vi "real time object finder single cam 4 way v2.1 EJA 09 19 2016.vi"() -> ()   [LabVIEW 2013]
doc: "The Low-Level Grab VI acquires images continuously and displays the images in an image control using low-level acquisition VIs. A grab is appropriate for high-speed applications in which you need to process only one image at a time."
uses:
  <vilib>/userdefined/High Color/IMAQdx.ctl
  <vilib>/vision/driver/IMAQdx.llb/IMAQdx Buffer Number Mode.ctl
  <vilib>/Utility/file.llb/Write To Spreadsheet File (I64).vi
  <vilib>/vision/driver/NI_Vision_Acquisition_Software.lvlib
  <resource>/objmgr/imaqdx.rc
  <vilib>/Analysis/NI_AALBase.lvlib
panel:
  in  "Rectangle":T1
  in  "fish size":i32=200
  out "y position histogram":T2(graph)={"X Values"=[445.05, 445.15, 445.25, 445.35, 445.45, 445.55, 445.65, 445.75, 445.85, 445.95], "Histogram: h(x)"=[229, 0, 0, 0, 0, 0, 0, 0, 0, 272]}
  out "x position histogram":T2(graph)={"X Values"=[585.0, 585.0, 585.0, 585.0, 585.0, 585.0, 585.0, 585.0, 585.0, 585.0], "Histogram: h(x)"=[0, 0, 0, 0, 0, 0, 0, 0, 0, 501]}
  in  "histogram \nbins":i32=10
  in  "always save\non stop\nimaging":bool=TRUE
  in  "acquisition \ntime (s)":i32=10
  in  "save for a \ndesignated \nperiod":bool=TRUE
  out "trajectory":cluster{i32[], i32[]}(graph)={[585, 585, 585, 585, 585, 585, 585, 585, 585, 585, 585, 585, 585, 585, 585, 585, 585, 585, 585, 585, 585, 585, 585, 585, 585, 585, 585, 585, 585, 585, 585, 585, 585, 585, 585, 585, 585, 585, 585, 585, 585, 585, 585, 585, 585, 585, 585, 585, 585, 585, 585, 585, 585, 585, 585, 585, 585, 585, 585, 585, 585, 585, 585, 585, 585, 585, 585, 585, 585, 585, 585, 585, 585, 585, 585, 585, 585, 585, 585, 585, 585, 585, 585, 585, 585, 585, 585, 585, 585, 585, 585, 585, 585, 585, 585, 585, 585, 585, 585, 585, 585, 585, 585, 585, 585, 585, 585, 585, 585, 585, 585, 585, 585, 585, 585, 585, 585, 585, 585, 585, 585, 585, 585, 585, 585, 585, 585, 585, 585, 585, 585, 585, 585, 585, 585, 585, 585, 585, 585, 585, 585, 585, 585, 585, 585, 585, 585, 585, 585, 585, 585, 585, 585, 585, 585, 585, 585, 585, 585, 585, 585, 585, 585, 585, 585, 585, 585, 585, 585, 585, 585, 585, 585, 585, 585, 585, 585, 585, 585, 585, 585, 585, 585, 585, 585, 585, 585, 585, 585, 585, 585, 585, 585, 585, 585, 585, 585, 585, 585, 585, 585, 585, 585, 585, 585, 585, 585, 585, 585, 585, 585, 585, 585, 585, 585, 585, 585, 585, 585, 585, 585, 585, 585, 585, 585, 585, 585, 585, 585, 585, 585, 585, 585, 585, 585, 585, 585, 585, 585, 585, 585, 585, 585, 585, 585, 585, 585, 585, 585, 585, 585, 585, 585, 585, 585, 585, 585, 585, 585, 585, 585, 585, 585, 585, 585, 585, 585, 585, 585, 585, 585, 585, 585, 585, 585, 585, 585, 585, 585, 585, 585, 585, 585, 585, 585, 585, 585, 585, 585, 585, 585, 585, 585, 585, 585, 585, 585, 585, 585, 585, 585, 585, 585, 585, 585, 585, 585, 585, 585, 585, 585, 585, 585, 585, 585, 585, 585, 585, 585, 585, 585, 585, 585, 585, 585, 585, 585, 585, 585, 585, 585, 585, 585, 585, 585, 585, 585, 585, 585, 585, 585, 585, 585, 585, 585, 585, 585, 585, 585, 585, 585, 585, 585, 585, 585, 585, 585, 585, 585, 585, 585, 585, 585, 585, 585, 585, 585, 585, 585, 585, 585, 585, 585, 585, 585, 585, 585, 585, 585, 585, 585, 585, 585, 585, 585, 585, 585, 585, 585, 585, 585, 585, 585, 585, 585, 585, 585, 585, 585, 585, 585, 585, 585, 585, 585, 585, 585, 585, 585, 585, 585, 585, 585, 585, 585, 585, 585, 585, 585, 585, 585, 585, 585, 585, 585, 585, 585, 585, 585, 585, 585, 585, 585, 585, 585, 585, 585, 585, 585, 585, 585, 585, 585, 585, 585, 585, 585, 585, 585, 585, 585, 585, 585, 585, 585, 585, 585, 585, 585, 585, 585, 585, 585, 585, 585, 585, 585, 585, 585, 585, 585, 585, 585, 585, 585, 585, 585, 585, 585, 585, 585, 585, 585, 585, 585, 585, 585, 585, 585, 585, 585, 585, 585, 585, 585, 585, 585, 585, 585, 585, 585], [446, 446, 446, 445, 446, 445, 446, 446, 446, 446, 446, 445, 445, 446, 445, 446, 445, 446, 446, 446, 445, 445, 446, 446, 445, 445, 446, 445, 446, 445, 445, 445, 445, 445, 446, 446, 445, 445, 445, 446, 446, 445, 445, 445, 446, 446, 446, 445, 446, 446, 446, 446, 446, 445, 446, 446, 445, 446, 445, 446, 445, 445, 445, 446, 445, 446, 446, 446, 446, 446, 445, 445, 445, 445, 446, 445, 445, 445, 445, 446, 445, 446, 446, 446, 446, 446, 446, 445, 445, 446, 445, 445, 445, 445, 445, 445, 445, 445, 446, 446, 446, 445, 446, 445, 446, 445, 445, 446, 446, 446, 446, 445, 446, 445, 446, 445, 445, 445, 446, 446, 445, 445, 446, 445, 446, 445, 446, 446, 445, 446, 446, 445, 445, 445, 446, 445, 446, 445, 445, 446, 446, 445, 445, 446, 445, 446, 446, 446, 446, 445, 445, 446, 445, 445, 446, 445, 445, 445, 445, 445, 445, 446, 446, 445, 446, 445, 446, 446, 445, 446, 445, 446, 446, 445, 446, 446, 445, 446, 445, 446, 446, 446, 445, 446, 445, 446, 446, 445, 446, 445, 446, 445, 446, 445, 446, 445, 445, 445, 446, 445, 446, 446, 446, 445, 445, 446, 446, 446, 445, 446, 445, 446, 445, 446, 446, 446, 446, 446, 446, 446, 446, 445, 446, 445, 445, 445, 446, 445, 445, 446, 445, 445, 446, 446, 446, 445, 446, 445, 446, 446, 446, 445, 445, 445, 446, 446, 446, 445, 445, 445, 446, 445, 445, 446, 445, 445, 446, 446, 445, 445, 446, 446, 446, 446, 446, 446, 446, 446, 446, 446, 445, 446, 445, 445, 445, 446, 445, 446, 445, 446, 445, 445, 445, 446, 446, 446, 445, 446, 445, 445, 445, 446, 446, 446, 446, 445, 446, 446, 446, 445, 445, 445, 446, 446, 446, 446, 445, 446, 445, 446, 446, 445, 446, 446, 446, 446, 445, 446, 445, 445, 445, 446, 446, 445, 446, 446, 445, 446, 446, 446, 446, 446, 446, 445, 446, 446, 445, 446, 446, 445, 446, 445, 446, 446, 446, 446, 445, 446, 446, 446, 446, 446, 445, 446, 446, 446, 446, 446, 446, 446, 445, 445, 445, 445, 445, 445, 445, 446, 445, 446, 446, 446, 446, 445, 446, 446, 445, 445, 445, 445, 445, 446, 445, 445, 445, 445, 446, 446, 445, 445, 445, 445, 446, 445, 446, 446, 446, 446, 445, 445, 445, 445, 445, 446, 445, 445, 446, 445, 445, 446, 446, 446, 445, 446, 445, 446, 445, 446, 445, 446, 445, 446, 445, 446, 446, 445, 446, 445, 446, 445, 445, 446, 446, 445, 445, 445, 445, 445, 446, 445, 445, 446, 446, 446, 446, 445, 446, 445, 446, 446, 446, 445, 445, 446, 445, 446, 446, 446, 446, 445, 446, 445, 446, 446, 445, 446, 446, 445, 445, 446, 446, 445, 446, 446, 446, 445, 446, 446, 446, 445, 445, 445, 446, 445, 446, 446, 446, 446, 445, 445, 446, 445, 445, 446, 445, 446, 446, 446, 446, 446, 445]}
  in  "save\nlast\nimage":bool=TRUE
  in  "stop no save":bool
  out "date stub assigned":string="_2016Y_10M_31D_13h_16m_16s"
  in  "Acquire\ndata":bool
  in  "Experimental stub":string="danio02"
  out "Saving":bool
  in  "save data":bool
  in  "save path":path=path "C:/danio_tracking/danio02_10_28_2016"
  in  "number\nformat (%.6f)":string="%.6f"
  in  "Marker\nText color":u32(colorbox)=16711680
  out "Multiplot":cluster{cluster{dbl, i32}[]}[](graph)=[{[{0.0, 585}, {0.02, 585}, {0.04, 585}, {0.06, 585}, {0.08, 585}, {0.1, 585}, {0.12, 585}, {0.14, 585}, {0.16, 585}, {0.18, 585}, {0.2, 585}, {0.22, 585}, {0.24, 585}, {0.26, 585}, {0.281, 585}, {0.301, 585}, {0.321, 585}, {0.341, 585}, {0.361, 585}, {0.382, 585}, {0.401, 585}, {0.421, 585}, {0.441, 585}, {0.461, 585}, {0.481, 585}, {0.501, 585}, {0.521, 585}, {0.541, 585}, {0.561, 585}, {0.582, 585}, {0.601, 585}, {0.621, 585}, {0.641, 585}, {0.661, 585}, {0.682, 585}, {0.702, 585}, {0.721, 585}, {0.741, 585}, {0.761, 585}, {0.782, 585}, {0.801, 585}, {0.821, 585}, {0.842, 585}, {0.862, 585}, {0.882, 585}, {0.901, 585}, {0.921, 585}, {0.941, 585}, {0.961, 585}, {0.982, 585}, {1.002, 585}, {1.022, 585}, {1.042, 585}, {1.062, 585}, {1.082, 585}, {1.102, 585}, {1.122, 585}, {1.142, 585}, {1.162, 585}, {1.182, 585}, {1.202, 585}, {1.222, 585}, {1.242, 585}, {1.262, 585}, {1.282, 585}, {1.302, 585}, {1.322, 585}, {1.342, 585}, {1.362, 585}, {1.382, 585}, {1.402, 585}, {1.422, 585}, {1.442, 585}, {1.462, 585}, {1.482, 585}, {1.502, 585}, {1.522, 585}, {1.542, 585}, {1.562, 585}, {1.582, 585}, {1.602, 585}, {1.622, 585}, {1.642, 585}, {1.662, 585}, {1.683, 585}, {1.703, 585}, {1.723, 585}, {1.743, 585}, {1.764, 585}, {1.783, 585}, {1.803, 585}, {1.823, 585}, {1.843, 585}, {1.863, 585}, {1.883, 585}, {1.903, 585}, {1.923, 585}, {1.943, 585}, {1.963, 585}, {1.984, 585}, {2.003, 585}, {2.023, 585}, {2.043, 585}, {2.064, 585}, {2.084, 585}, {2.104, 585}, {2.124, 585}, {2.144, 585}, {2.164, 585}, {2.184, 585}, {2.204, 585}, {2.224, 585}, {2.244, 585}, {2.264, 585}, {2.284, 585}, {2.304, 585}, {2.324, 585}, {2.344, 585}, {2.364, 585}, {2.384, 585}, {2.404, 585}, {2.424, 585}, {2.444, 585}, {2.464, 585}, {2.484, 585}, {2.504, 585}, {2.524, 585}, {2.544, 585}, {2.564, 585}, {2.584, 585}, {2.604, 585}, {2.624, 585}, {2.644, 585}, {2.664, 585}, {2.684, 585}, {2.704, 585}, {2.724, 585}, {2.744, 585}, {2.764, 585}, {2.784, 585}, {2.804, 585}, {2.824, 585}, {2.844, 585}, {2.864, 585}, {2.884, 585}, {2.904, 585}, {2.924, 585}, {2.944, 585}, {2.964, 585}, {2.984, 585}, {3.004, 585}, {3.024, 585}, {3.044, 585}, {3.064, 585}, {3.084, 585}, {3.104, 585}, {3.126, 585}, {3.146, 585}, {3.166, 585}, {3.186, 585}, {3.206, 585}, {3.226, 585}, {3.246, 585}, {3.266, 585}, {3.286, 585}, {3.306, 585}, {3.326, 585}, {3.346, 585}, {3.366, 585}, {3.386, 585}, {3.406, 585}, {3.426, 585}, {3.446, 585}, {3.466, 585}, {3.486, 585}, {3.506, 585}, {3.526, 585}, {3.546, 585}, {3.566, 585}, {3.586, 585}, {3.606, 585}, {3.626, 585}, {3.646, 585}, {3.666, 585}, {3.686, 585}, {3.706, 585}, {3.726, 585}, {3.746, 585}, {3.767, 585}, {3.786, 585}, {3.806, 585}, {3.826, 585}, {3.846, 585}, {3.867, 585}, {3.886, 585}, {3.906, 585}, {3.926, 585}, {3.946, 585}, {3.967, 585}, {3.986, 585}, {4.006, 585}, {4.026, 585}, {4.046, 585}, {4.067, 585}, {4.086, 585}, {4.106, 585}, {4.126, 585}, {4.146, 585}, {4.167, 585}, {4.186, 585}, {4.206, 585}, {4.226, 585}, {4.246, 585}, {4.267, 585}, {4.287, 585}, {4.307, 585}, {4.327, 585}, {4.347, 585}, {4.367, 585}, {4.387, 585}, {4.407, 585}, {4.427, 585}, {4.447, 585}, {4.467, 585}, {4.488, 585}, {4.507, 585}, {4.528, 585}, {4.548, 585}, {4.568, 585}, {4.588, 585}, {4.608, 585}, {4.628, 585}, {4.648, 585}, {4.668, 585}, {4.688, 585}, {4.708, 585}, {4.728, 585}, {4.748, 585}, {4.768, 585}, {4.788, 585}, {4.808, 585}, {4.828, 585}, {4.848, 585}, {4.868, 585}, {4.888, 585}, {4.908, 585}, {4.928, 585}, {4.948, 585}, {4.968, 585}, {4.988, 585}, {5.008, 585}, {5.028, 585}, {5.048, 585}, {5.069, 585}, {5.088, 585}, {5.108, 585}, {5.128, 585}, {5.148, 585}, {5.169, 585}, {5.188, 585}, {5.208, 585}, {5.228, 585}, {5.248, 585}, {5.268, 585}, {5.288, 585}, {5.308, 585}, {5.329, 585}, {5.348, 585}, {5.369, 585}, {5.389, 585}, {5.409, 585}, {5.429, 585}, {5.449, 585}, {5.469, 585}, {5.489, 585}, {5.509, 585}, {5.529, 585}, {5.549, 585}, {5.569, 585}, {5.589, 585}, {5.609, 585}, {5.629, 585}, {5.649, 585}, {5.669, 585}, {5.689, 585}, {5.709, 585}, {5.729, 585}, {5.749, 585}, {5.769, 585}, {5.789, 585}, {5.809, 585}, {5.829, 585}, {5.849, 585}, {5.869, 585}, {5.889, 585}, {5.909, 585}, {5.93, 585}, {5.95, 585}, {5.97, 585}, {5.99, 585}, {6.01, 585}, {6.03, 585}, {6.05, 585}, {6.07, 585}, {6.09, 585}, {6.11, 585}, {6.13, 585}, {6.15, 585}, {6.17, 585}, {6.19, 585}, {6.21, 585}, {6.23, 585}, {6.25, 585}, {6.27, 585}, {6.29, 585}, {6.311, 585}, {6.33, 585}, {6.35, 585}, {6.37, 585}, {6.39, 585}, {6.411, 585}, {6.431, 585}, {6.45, 585}, {6.471, 585}, {6.491, 585}, {6.511, 585}, {6.531, 585}, {6.551, 585}, {6.571, 585}, {6.591, 585}, {6.611, 585}, {6.631, 585}, {6.651, 585}, {6.671, 585}, {6.691, 585}, {6.711, 585}, {6.731, 585}, {6.751, 585}, {6.771, 585}, {6.791, 585}, {6.811, 585}, {6.831, 585}, {6.852, 585}, {6.871, 585}, {6.891, 585}, {6.911, 585}, {6.931, 585}, {6.951, 585}, {6.971, 585}, {6.991, 585}, {7.011, 585}, {7.031, 585}, {7.051, 585}, {7.071, 585}, {7.091, 585}, {7.111, 585}, {7.131, 585}, {7.151, 585}, {7.171, 585}, {7.191, 585}, {7.211, 585}, {7.231, 585}, {7.252, 585}, {7.271, 585}, {7.291, 585}, {7.311, 585}, {7.332, 585}, {7.353, 585}, {7.372, 585}, {7.392, 585}, {7.412, 585}, {7.432, 585}, {7.453, 585}, {7.472, 585}, {7.492, 585}, {7.513, 585}, {7.532, 585}, {7.553, 585}, {7.573, 585}, {7.593, 585}, {7.613, 585}, {7.633, 585}, {7.653, 585}, {7.673, 585}, {7.693, 585}, {7.713, 585}, {7.733, 585}, {7.753, 585}, {7.773, 585}, {7.793, 585}, {7.813, 585}, {7.833, 585}, {7.853, 585}, {7.873, 585}, {7.893, 585}, {7.913, 585}, {7.933, 585}, {7.954, 585}, {7.973, 585}, {7.993, 585}, {8.013, 585}, {8.033, 585}, {8.053, 585}, {8.073, 585}, {8.093, 585}, {8.113, 585}, {8.133, 585}, {8.154, 585}, {8.173, 585}, {8.193, 585}, {8.213, 585}, {8.233, 585}, {8.254, 585}, {8.273, 585}, {8.293, 585}, {8.313, 585}, {8.333, 585}, {8.353, 585}, {8.373, 585}, {8.393, 585}, {8.413, 585}, {8.433, 585}, {8.454, 585}, {8.473, 585}, {8.493, 585}, {8.513, 585}, {8.533, 585}, {8.554, 585}, {8.574, 585}, {8.594, 585}, {8.614, 585}, {8.634, 585}, {8.654, 585}, {8.674, 585}, {8.694, 585}, {8.714, 585}, {8.735, 585}, {8.755, 585}, {8.775, 585}, {8.795, 585}, {8.815, 585}, {8.835, 585}, {8.855, 585}, {8.875, 585}, {8.895, 585}, {8.915, 585}, {8.935, 585}, {8.955, 585}, {8.975, 585}, {8.995, 585}, {9.015, 585}, {9.035, 585}, {9.055, 585}, {9.075, 585}, {9.095, 585}, {9.115, 585}, {9.135, 585}, {9.155, 585}, {9.175, 585}, {9.195, 585}, {9.215, 585}, {9.235, 585}, {9.255, 585}, {9.275, 585}, {9.295, 585}, {9.315, 585}, {9.335, 585}, {9.355, 585}, {9.375, 585}, {9.395, 585}, {9.415, 585}, {9.435, 585}, {9.456, 585}, {9.475, 585}, {9.495, 585}, {9.515, 585}, {9.535, 585}, {9.555, 585}, {9.576, 585}, {9.595, 585}, {9.615, 585}, {9.636, 585}, {9.655, 585}, {9.675, 585}, {9.696, 585}, {9.716, 585}, {9.736, 585}, {9.755, 585}, {9.776, 585}, {9.796, 585}, {9.816, 585}, {9.836, 585}, {9.856, 585}, {9.876, 585}, {9.896, 585}, {9.916, 585}, {9.936, 585}, {9.956, 585}, {9.976, 585}, {9.996, 585}, {10.016, 585}]}, {[{0.0, 446}, {0.02, 446}, {0.04, 446}, {0.06, 445}, {0.08, 446}, {0.1, 445}, {0.12, 446}, {0.14, 446}, {0.16, 446}, {0.18, 446}, {0.2, 446}, {0.22, 445}, {0.24, 445}, {0.26, 446}, {0.281, 445}, {0.301, 446}, {0.321, 445}, {0.341, 446}, {0.361, 446}, {0.382, 446}, {0.401, 445}, {0.421, 445}, {0.441, 446}, {0.461, 446}, {0.481, 445}, {0.501, 445}, {0.521, 446}, {0.541, 445}, {0.561, 446}, {0.582, 445}, {0.601, 445}, {0.621, 445}, {0.641, 445}, {0.661, 445}, {0.682, 446}, {0.702, 446}, {0.721, 445}, {0.741, 445}, {0.761, 445}, {0.782, 446}, {0.801, 446}, {0.821, 445}, {0.842, 445}, {0.862, 445}, {0.882, 446}, {0.901, 446}, {0.921, 446}, {0.941, 445}, {0.961, 446}, {0.982, 446}, {1.002, 446}, {1.022, 446}, {1.042, 446}, {1.062, 445}, {1.082, 446}, {1.102, 446}, {1.122, 445}, {1.142, 446}, {1.162, 445}, {1.182, 446}, {1.202, 445}, {1.222, 445}, {1.242, 445}, {1.262, 446}, {1.282, 445}, {1.302, 446}, {1.322, 446}, {1.342, 446}, {1.362, 446}, {1.382, 446}, {1.402, 445}, {1.422, 445}, {1.442, 445}, {1.462, 445}, {1.482, 446}, {1.502, 445}, {1.522, 445}, {1.542, 445}, {1.562, 445}, {1.582, 446}, {1.602, 445}, {1.622, 446}, {1.642, 446}, {1.662, 446}, {1.683, 446}, {1.703, 446}, {1.723, 446}, {1.743, 445}, {1.764, 445}, {1.783, 446}, {1.803, 445}, {1.823, 445}, {1.843, 445}, {1.863, 445}, {1.883, 445}, {1.903, 445}, {1.923, 445}, {1.943, 445}, {1.963, 446}, {1.984, 446}, {2.003, 446}, {2.023, 445}, {2.043, 446}, {2.064, 445}, {2.084, 446}, {2.104, 445}, {2.124, 445}, {2.144, 446}, {2.164, 446}, {2.184, 446}, {2.204, 446}, {2.224, 445}, {2.244, 446}, {2.264, 445}, {2.284, 446}, {2.304, 445}, {2.324, 445}, {2.344, 445}, {2.364, 446}, {2.384, 446}, {2.404, 445}, {2.424, 445}, {2.444, 446}, {2.464, 445}, {2.484, 446}, {2.504, 445}, {2.524, 446}, {2.544, 446}, {2.564, 445}, {2.584, 446}, {2.604, 446}, {2.624, 445}, {2.644, 445}, {2.664, 445}, {2.684, 446}, {2.704, 445}, {2.724, 446}, {2.744, 445}, {2.764, 445}, {2.784, 446}, {2.804, 446}, {2.824, 445}, {2.844, 445}, {2.864, 446}, {2.884, 445}, {2.904, 446}, {2.924, 446}, {2.944, 446}, {2.964, 446}, {2.984, 445}, {3.004, 445}, {3.024, 446}, {3.044, 445}, {3.064, 445}, {3.084, 446}, {3.104, 445}, {3.126, 445}, {3.146, 445}, {3.166, 445}, {3.186, 445}, {3.206, 445}, {3.226, 446}, {3.246, 446}, {3.266, 445}, {3.286, 446}, {3.306, 445}, {3.326, 446}, {3.346, 446}, {3.366, 445}, {3.386, 446}, {3.406, 445}, {3.426, 446}, {3.446, 446}, {3.466, 445}, {3.486, 446}, {3.506, 446}, {3.526, 445}, {3.546, 446}, {3.566, 445}, {3.586, 446}, {3.606, 446}, {3.626, 446}, {3.646, 445}, {3.666, 446}, {3.686, 445}, {3.706, 446}, {3.726, 446}, {3.746, 445}, {3.767, 446}, {3.786, 445}, {3.806, 446}, {3.826, 445}, {3.846, 446}, {3.867, 445}, {3.886, 446}, {3.906, 445}, {3.926, 445}, {3.946, 445}, {3.967, 446}, {3.986, 445}, {4.006, 446}, {4.026, 446}, {4.046, 446}, {4.067, 445}, {4.086, 445}, {4.106, 446}, {4.126, 446}, {4.146, 446}, {4.167, 445}, {4.186, 446}, {4.206, 445}, {4.226, 446}, {4.246, 445}, {4.267, 446}, {4.287, 446}, {4.307, 446}, {4.327, 446}, {4.347, 446}, {4.367, 446}, {4.387, 446}, {4.407, 446}, {4.427, 445}, {4.447, 446}, {4.467, 445}, {4.488, 445}, {4.507, 445}, {4.528, 446}, {4.548, 445}, {4.568, 445}, {4.588, 446}, {4.608, 445}, {4.628, 445}, {4.648, 446}, {4.668, 446}, {4.688, 446}, {4.708, 445}, {4.728, 446}, {4.748, 445}, {4.768, 446}, {4.788, 446}, {4.808, 446}, {4.828, 445}, {4.848, 445}, {4.868, 445}, {4.888, 446}, {4.908, 446}, {4.928, 446}, {4.948, 445}, {4.968, 445}, {4.988, 445}, {5.008, 446}, {5.028, 445}, {5.048, 445}, {5.069, 446}, {5.088, 445}, {5.108, 445}, {5.128, 446}, {5.148, 446}, {5.169, 445}, {5.188, 445}, {5.208, 446}, {5.228, 446}, {5.248, 446}, {5.268, 446}, {5.288, 446}, {5.308, 446}, {5.329, 446}, {5.348, 446}, {5.369, 446}, {5.389, 446}, {5.409, 445}, {5.429, 446}, {5.449, 445}, {5.469, 445}, {5.489, 445}, {5.509, 446}, {5.529, 445}, {5.549, 446}, {5.569, 445}, {5.589, 446}, {5.609, 445}, {5.629, 445}, {5.649, 445}, {5.669, 446}, {5.689, 446}, {5.709, 446}, {5.729, 445}, {5.749, 446}, {5.769, 445}, {5.789, 445}, {5.809, 445}, {5.829, 446}, {5.849, 446}, {5.869, 446}, {5.889, 446}, {5.909, 445}, {5.93, 446}, {5.95, 446}, {5.97, 446}, {5.99, 445}, {6.01, 445}, {6.03, 445}, {6.05, 446}, {6.07, 446}, {6.09, 446}, {6.11, 446}, {6.13, 445}, {6.15, 446}, {6.17, 445}, {6.19, 446}, {6.21, 446}, {6.23, 445}, {6.25, 446}, {6.27, 446}, {6.29, 446}, {6.311, 446}, {6.33, 445}, {6.35, 446}, {6.37, 445}, {6.39, 445}, {6.411, 445}, {6.431, 446}, {6.45, 446}, {6.471, 445}, {6.491, 446}, {6.511, 446}, {6.531, 445}, {6.551, 446}, {6.571, 446}, {6.591, 446}, {6.611, 446}, {6.631, 446}, {6.651, 446}, {6.671, 445}, {6.691, 446}, {6.711, 446}, {6.731, 445}, {6.751, 446}, {6.771, 446}, {6.791, 445}, {6.811, 446}, {6.831, 445}, {6.852, 446}, {6.871, 446}, {6.891, 446}, {6.911, 446}, {6.931, 445}, {6.951, 446}, {6.971, 446}, {6.991, 446}, {7.011, 446}, {7.031, 446}, {7.051, 445}, {7.071, 446}, {7.091, 446}, {7.111, 446}, {7.131, 446}, {7.151, 446}, {7.171, 446}, {7.191, 446}, {7.211, 445}, {7.231, 445}, {7.252, 445}, {7.271, 445}, {7.291, 445}, {7.311, 445}, {7.332, 445}, {7.353, 446}, {7.372, 445}, {7.392, 446}, {7.412, 446}, {7.432, 446}, {7.453, 446}, {7.472, 445}, {7.492, 446}, {7.513, 446}, {7.532, 445}, {7.553, 445}, {7.573, 445}, {7.593, 445}, {7.613, 445}, {7.633, 446}, {7.653, 445}, {7.673, 445}, {7.693, 445}, {7.713, 445}, {7.733, 446}, {7.753, 446}, {7.773, 445}, {7.793, 445}, {7.813, 445}, {7.833, 445}, {7.853, 446}, {7.873, 445}, {7.893, 446}, {7.913, 446}, {7.933, 446}, {7.954, 446}, {7.973, 445}, {7.993, 445}, {8.013, 445}, {8.033, 445}, {8.053, 445}, {8.073, 446}, {8.093, 445}, {8.113, 445}, {8.133, 446}, {8.154, 445}, {8.173, 445}, {8.193, 446}, {8.213, 446}, {8.233, 446}, {8.254, 445}, {8.273, 446}, {8.293, 445}, {8.313, 446}, {8.333, 445}, {8.353, 446}, {8.373, 445}, {8.393, 446}, {8.413, 445}, {8.433, 446}, {8.454, 445}, {8.473, 446}, {8.493, 446}, {8.513, 445}, {8.533, 446}, {8.554, 445}, {8.574, 446}, {8.594, 445}, {8.614, 445}, {8.634, 446}, {8.654, 446}, {8.674, 445}, {8.694, 445}, {8.714, 445}, {8.735, 445}, {8.755, 445}, {8.775, 446}, {8.795, 445}, {8.815, 445}, {8.835, 446}, {8.855, 446}, {8.875, 446}, {8.895, 446}, {8.915, 445}, {8.935, 446}, {8.955, 445}, {8.975, 446}, {8.995, 446}, {9.015, 446}, {9.035, 445}, {9.055, 445}, {9.075, 446}, {9.095, 445}, {9.115, 446}, {9.135, 446}, {9.155, 446}, {9.175, 446}, {9.195, 445}, {9.215, 446}, {9.235, 445}, {9.255, 446}, {9.275, 446}, {9.295, 445}, {9.315, 446}, {9.335, 446}, {9.355, 445}, {9.375, 445}, {9.395, 446}, {9.415, 446}, {9.435, 445}, {9.456, 446}, {9.475, 446}, {9.495, 446}, {9.515, 445}, {9.535, 446}, {9.555, 446}, {9.576, 446}, {9.595, 445}, {9.615, 445}, {9.636, 445}, {9.655, 446}, {9.675, 445}, {9.696, 446}, {9.716, 446}, {9.736, 446}, {9.755, 446}, {9.776, 445}, {9.796, 445}, {9.816, 446}, {9.836, 445}, {9.856, 445}, {9.876, 446}, {9.896, 445}, {9.916, 446}, {9.936, 446}, {9.956, 446}, {9.976, 446}, {9.996, 446}, {10.016, 445}]}]
  out "FPS":i32=50
  out "time (s)":dbl[](array[numeric])=[0.0, 0.02, 0.04, 0.06, 0.08, 0.1, 0.12, 0.14, 0.16, 0.18, 0.2, 0.22, 0.24, 0.26, 0.281, 0.301, 0.321, 0.341, 0.361, 0.382, 0.401, 0.421, 0.441, 0.461, 0.481, 0.501, 0.521, 0.541, 0.561, 0.582, 0.601, 0.621, 0.641, 0.661, 0.682, 0.702, 0.721, 0.741, 0.761, 0.782, 0.801, 0.821, 0.842, 0.862, 0.882, 0.901, 0.921, 0.941, 0.961, 0.982, 1.002, 1.022, 1.042, 1.062, 1.082, 1.102, 1.122, 1.142, 1.162, 1.182, 1.202, 1.222, 1.242, 1.262, 1.282, 1.302, 1.322, 1.342, 1.362, 1.382, 1.402, 1.422, 1.442, 1.462, 1.482, 1.502, 1.522, 1.542, 1.562, 1.582, 1.602, 1.622, 1.642, 1.662, 1.683, 1.703, 1.723, 1.743, 1.764, 1.783, 1.803, 1.823, 1.843, 1.863, 1.883, 1.903, 1.923, 1.943, 1.963, 1.984, 2.003, 2.023, 2.043, 2.064, 2.084, 2.104, 2.124, 2.144, 2.164, 2.184, 2.204, 2.224, 2.244, 2.264, 2.284, 2.304, 2.324, 2.344, 2.364, 2.384, 2.404, 2.424, 2.444, 2.464, 2.484, 2.504, 2.524, 2.544, 2.564, 2.584, 2.604, 2.624, 2.644, 2.664, 2.684, 2.704, 2.724, 2.744, 2.764, 2.784, 2.804, 2.824, 2.844, 2.864, 2.884, 2.904, 2.924, 2.944, 2.964, 2.984, 3.004, 3.024, 3.044, 3.064, 3.084, 3.104, 3.126, 3.146, 3.166, 3.186, 3.206, 3.226, 3.246, 3.266, 3.286, 3.306, 3.326, 3.346, 3.366, 3.386, 3.406, 3.426, 3.446, 3.466, 3.486, 3.506, 3.526, 3.546, 3.566, 3.586, 3.606, 3.626, 3.646, 3.666, 3.686, 3.706, 3.726, 3.746, 3.767, 3.786, 3.806, 3.826, 3.846, 3.867, 3.886, 3.906, 3.926, 3.946, 3.967, 3.986, 4.006, 4.026, 4.046, 4.067, 4.086, 4.106, 4.126, 4.146, 4.167, 4.186, 4.206, 4.226, 4.246, 4.267, 4.287, 4.307, 4.327, 4.347, 4.367, 4.387, 4.407, 4.427, 4.447, 4.467, 4.488, 4.507, 4.528, 4.548, 4.568, 4.588, 4.608, 4.628, 4.648, 4.668, 4.688, 4.708, 4.728, 4.748, 4.768, 4.788, 4.808, 4.828, 4.848, 4.868, 4.888, 4.908, 4.928, 4.948, 4.968, 4.988, 5.008, 5.028, 5.048, 5.069, 5.088, 5.108, 5.128, 5.148, 5.169, 5.188, 5.208, 5.228, 5.248, 5.268, 5.288, 5.308, 5.329, 5.348, 5.369, 5.389, 5.409, 5.429, 5.449, 5.469, 5.489, 5.509, 5.529, 5.549, 5.569, 5.589, 5.609, 5.629, 5.649, 5.669, 5.689, 5.709, 5.729, 5.749, 5.769, 5.789, 5.809, 5.829, 5.849, 5.869, 5.889, 5.909, 5.93, 5.95, 5.97, 5.99, 6.01, 6.03, 6.05, 6.07, 6.09, 6.11, 6.13, 6.15, 6.17, 6.19, 6.21, 6.23, 6.25, 6.27, 6.29, 6.311, 6.33, 6.35, 6.37, 6.39, 6.411, 6.431, 6.45, 6.471, 6.491, 6.511, 6.531, 6.551, 6.571, 6.591, 6.611, 6.631, 6.651, 6.671, 6.691, 6.711, 6.731, 6.751, 6.771, 6.791, 6.811, 6.831, 6.852, 6.871, 6.891, 6.911, 6.931, 6.951, 6.971, 6.991, 7.011, 7.031, 7.051, 7.071, 7.091, 7.111, 7.131, 7.151, 7.171, 7.191, 7.211, 7.231, 7.252, 7.271, 7.291, 7.311, 7.332, 7.353, 7.372, 7.392, 7.412, 7.432, 7.453, 7.472, 7.492, 7.513, 7.532, 7.553, 7.573, 7.593, 7.613, 7.633, 7.653, 7.673, 7.693, 7.713, 7.733, 7.753, 7.773, 7.793, 7.813, 7.833, 7.853, 7.873, 7.893, 7.913, 7.933, 7.954, 7.973, 7.993, 8.013, 8.033, 8.053, 8.073, 8.093, 8.113, 8.133, 8.154, 8.173, 8.193, 8.213, 8.233, 8.254, 8.273, 8.293, 8.313, 8.333, 8.353, 8.373, 8.393, 8.413, 8.433, 8.454, 8.473, 8.493, 8.513, 8.533, 8.554, 8.574, 8.594, 8.614, 8.634, 8.654, 8.674, 8.694, 8.714, 8.735, 8.755, 8.775, 8.795, 8.815, 8.835, 8.855, 8.875, 8.895, 8.915, 8.935, 8.955, 8.975, 8.995, 9.015, 9.035, 9.055, 9.075, 9.095, 9.115, 9.135, 9.155, 9.175, 9.195, 9.215, 9.235, 9.255, 9.275, 9.295, 9.315, 9.335, 9.355, 9.375, 9.395, 9.415, 9.435, 9.456, 9.475, 9.495, 9.515, 9.535, 9.555, 9.576, 9.595, 9.615, 9.636, 9.655, 9.675, 9.696, 9.716, 9.736, 9.755, 9.776, 9.796, 9.816, 9.836, 9.856, 9.876, 9.896, 9.916, 9.936, 9.956, 9.976, 9.996, 10.016] format="%.3f"
  in  "Origin":cluster{"X":i32, "Y":i32}
  out "Y position vs time":cluster{dbl[], i32[]}(graph)={array[501 elements], [446, 446, 446, 445, 446, 445, 446, 446, 446, 446, 446, 445, 445, 446, 445, 446, 445, 446, 446, 446, 445, 445, 446, 446, 445, 445, 446, 445, 446, 445, 445, 445, 445, 445, 446, 446, 445, 445, 445, 446, 446, 445, 445, 445, 446, 446, 446, 445, 446, 446, 446, 446, 446, 445, 446, 446, 445, 446, 445, 446, 445, 445, 445, 446, 445, 446, 446, 446, 446, 446, 445, 445, 445, 445, 446, 445, 445, 445, 445, 446, 445, 446, 446, 446, 446, 446, 446, 445, 445, 446, 445, 445, 445, 445, 445, 445, 445, 445, 446, 446, 446, 445, 446, 445, 446, 445, 445, 446, 446, 446, 446, 445, 446, 445, 446, 445, 445, 445, 446, 446, 445, 445, 446, 445, 446, 445, 446, 446, 445, 446, 446, 445, 445, 445, 446, 445, 446, 445, 445, 446, 446, 445, 445, 446, 445, 446, 446, 446, 446, 445, 445, 446, 445, 445, 446, 445, 445, 445, 445, 445, 445, 446, 446, 445, 446, 445, 446, 446, 445, 446, 445, 446, 446, 445, 446, 446, 445, 446, 445, 446, 446, 446, 445, 446, 445, 446, 446, 445, 446, 445, 446, 445, 446, 445, 446, 445, 445, 445, 446, 445, 446, 446, 446, 445, 445, 446, 446, 446, 445, 446, 445, 446, 445, 446, 446, 446, 446, 446, 446, 446, 446, 445, 446, 445, 445, 445, 446, 445, 445, 446, 445, 445, 446, 446, 446, 445, 446, 445, 446, 446, 446, 445, 445, 445, 446, 446, 446, 445, 445, 445, 446, 445, 445, 446, 445, 445, 446, 446, 445, 445, 446, 446, 446, 446, 446, 446, 446, 446, 446, 446, 445, 446, 445, 445, 445, 446, 445, 446, 445, 446, 445, 445, 445, 446, 446, 446, 445, 446, 445, 445, 445, 446, 446, 446, 446, 445, 446, 446, 446, 445, 445, 445, 446, 446, 446, 446, 445, 446, 445, 446, 446, 445, 446, 446, 446, 446, 445, 446, 445, 445, 445, 446, 446, 445, 446, 446, 445, 446, 446, 446, 446, 446, 446, 445, 446, 446, 445, 446, 446, 445, 446, 445, 446, 446, 446, 446, 445, 446, 446, 446, 446, 446, 445, 446, 446, 446, 446, 446, 446, 446, 445, 445, 445, 445, 445, 445, 445, 446, 445, 446, 446, 446, 446, 445, 446, 446, 445, 445, 445, 445, 445, 446, 445, 445, 445, 445, 446, 446, 445, 445, 445, 445, 446, 445, 446, 446, 446, 446, 445, 445, 445, 445, 445, 446, 445, 445, 446, 445, 445, 446, 446, 446, 445, 446, 445, 446, 445, 446, 445, 446, 445, 446, 445, 446, 446, 445, 446, 445, 446, 445, 445, 446, 446, 445, 445, 445, 445, 445, 446, 445, 445, 446, 446, 446, 446, 445, 446, 445, 446, 446, 446, 445, 445, 446, 445, 446, 446, 446, 446, 445, 446, 445, 446, 446, 445, 446, 446, 445, 445, 446, 446, 445, 446, 446, 446, 445, 446, 446, 446, 445, 445, 445, 446, 445, 446, 446, 446, 446, 445, 445, 446, 445, 445, 446, 445, 446, 446, 446, 446, 446, 445]}
  out "X position vs time":cluster{dbl[], i32[]}(graph)={array[501 elements], [585, 585, 585, 585, 585, 585, 585, 585, 585, 585, 585, 585, 585, 585, 585, 585, 585, 585, 585, 585, 585, 585, 585, 585, 585, 585, 585, 585, 585, 585, 585, 585, 585, 585, 585, 585, 585, 585, 585, 585, 585, 585, 585, 585, 585, 585, 585, 585, 585, 585, 585, 585, 585, 585, 585, 585, 585, 585, 585, 585, 585, 585, 585, 585, 585, 585, 585, 585, 585, 585, 585, 585, 585, 585, 585, 585, 585, 585, 585, 585, 585, 585, 585, 585, 585, 585, 585, 585, 585, 585, 585, 585, 585, 585, 585, 585, 585, 585, 585, 585, 585, 585, 585, 585, 585, 585, 585, 585, 585, 585, 585, 585, 585, 585, 585, 585, 585, 585, 585, 585, 585, 585, 585, 585, 585, 585, 585, 585, 585, 585, 585, 585, 585, 585, 585, 585, 585, 585, 585, 585, 585, 585, 585, 585, 585, 585, 585, 585, 585, 585, 585, 585, 585, 585, 585, 585, 585, 585, 585, 585, 585, 585, 585, 585, 585, 585, 585, 585, 585, 585, 585, 585, 585, 585, 585, 585, 585, 585, 585, 585, 585, 585, 585, 585, 585, 585, 585, 585, 585, 585, 585, 585, 585, 585, 585, 585, 585, 585, 585, 585, 585, 585, 585, 585, 585, 585, 585, 585, 585, 585, 585, 585, 585, 585, 585, 585, 585, 585, 585, 585, 585, 585, 585, 585, 585, 585, 585, 585, 585, 585, 585, 585, 585, 585, 585, 585, 585, 585, 585, 585, 585, 585, 585, 585, 585, 585, 585, 585, 585, 585, 585, 585, 585, 585, 585, 585, 585, 585, 585, 585, 585, 585, 585, 585, 585, 585, 585, 585, 585, 585, 585, 585, 585, 585, 585, 585, 585, 585, 585, 585, 585, 585, 585, 585, 585, 585, 585, 585, 585, 585, 585, 585, 585, 585, 585, 585, 585, 585, 585, 585, 585, 585, 585, 585, 585, 585, 585, 585, 585, 585, 585, 585, 585, 585, 585, 585, 585, 585, 585, 585, 585, 585, 585, 585, 585, 585, 585, 585, 585, 585, 585, 585, 585, 585, 585, 585, 585, 585, 585, 585, 585, 585, 585, 585, 585, 585, 585, 585, 585, 585, 585, 585, 585, 585, 585, 585, 585, 585, 585, 585, 585, 585, 585, 585, 585, 585, 585, 585, 585, 585, 585, 585, 585, 585, 585, 585, 585, 585, 585, 585, 585, 585, 585, 585, 585, 585, 585, 585, 585, 585, 585, 585, 585, 585, 585, 585, 585, 585, 585, 585, 585, 585, 585, 585, 585, 585, 585, 585, 585, 585, 585, 585, 585, 585, 585, 585, 585, 585, 585, 585, 585, 585, 585, 585, 585, 585, 585, 585, 585, 585, 585, 585, 585, 585, 585, 585, 585, 585, 585, 585, 585, 585, 585, 585, 585, 585, 585, 585, 585, 585, 585, 585, 585, 585, 585, 585, 585, 585, 585, 585, 585, 585, 585, 585, 585, 585, 585, 585, 585, 585, 585, 585, 585, 585, 585, 585, 585, 585, 585, 585, 585, 585, 585, 585, 585, 585, 585, 585, 585, 585, 585, 585, 585, 585, 585, 585, 585, 585, 585, 585, 585]}
  in  "Pixel intensity\nthreshold":i32=65
  in  "Row min":i32=136
  in  "Row max":i32=630
  in  "Column min":i32=120
  in  "Column max":i32=1027
  out "X positions\ncamera 1\n(image \ncoordinates)":i32[](array[numeric])=[585, 585, 585, 585, 585, 585, 585, 585, 585, 585, 585, 585, 585, 585, 585, 585, 585, 585, 585, 585, 585, 585, 585, 585, 585, 585, 585, 585, 585, 585, 585, 585, 585, 585, 585, 585, 585, 585, 585, 585, 585, 585, 585, 585, 585, 585, 585, 585, 585, 585, 585, 585, 585, 585, 585, 585, 585, 585, 585, 585, 585, 585, 585, 585, 585, 585, 585, 585, 585, 585, 585, 585, 585, 585, 585, 585, 585, 585, 585, 585, 585, 585, 585, 585, 585, 585, 585, 585, 585, 585, 585, 585, 585, 585, 585, 585, 585, 585, 585, 585, 585, 585, 585, 585, 585, 585, 585, 585, 585, 585, 585, 585, 585, 585, 585, 585, 585, 585, 585, 585, 585, 585, 585, 585, 585, 585, 585, 585, 585, 585, 585, 585, 585, 585, 585, 585, 585, 585, 585, 585, 585, 585, 585, 585, 585, 585, 585, 585, 585, 585, 585, 585, 585, 585, 585, 585, 585, 585, 585, 585, 585, 585, 585, 585, 585, 585, 585, 585, 585, 585, 585, 585, 585, 585, 585, 585, 585, 585, 585, 585, 585, 585, 585, 585, 585, 585, 585, 585, 585, 585, 585, 585, 585, 585, 585, 585, 585, 585, 585, 585, 585, 585, 585, 585, 585, 585, 585, 585, 585, 585, 585, 585, 585, 585, 585, 585, 585, 585, 585, 585, 585, 585, 585, 585, 585, 585, 585, 585, 585, 585, 585, 585, 585, 585, 585, 585, 585, 585, 585, 585, 585, 585, 585, 585, 585, 585, 585, 585, 585, 585, 585, 585, 585, 585, 585, 585, 585, 585, 585, 585, 585, 585, 585, 585, 585, 585, 585, 585, 585, 585, 585, 585, 585, 585, 585, 585, 585, 585, 585, 585, 585, 585, 585, 585, 585, 585, 585, 585, 585, 585, 585, 585, 585, 585, 585, 585, 585, 585, 585, 585, 585, 585, 585, 585, 585, 585, 585, 585, 585, 585, 585, 585, 585, 585, 585, 585, 585, 585, 585, 585, 585, 585, 585, 585, 585, 585, 585, 585, 585, 585, 585, 585, 585, 585, 585, 585, 585, 585, 585, 585, 585, 585, 585, 585, 585, 585, 585, 585, 585, 585, 585, 585, 585, 585, 585, 585, 585, 585, 585, 585, 585, 585, 585, 585, 585, 585, 585, 585, 585, 585, 585, 585, 585, 585, 585, 585, 585, 585, 585, 585, 585, 585, 585, 585, 585, 585, 585, 585, 585, 585, 585, 585, 585, 585, 585, 585, 585, 585, 585, 585, 585, 585, 585, 585, 585, 585, 585, 585, 585, 585, 585, 585, 585, 585, 585, 585, 585, 585, 585, 585, 585, 585, 585, 585, 585, 585, 585, 585, 585, 585, 585, 585, 585, 585, 585, 585, 585, 585, 585, 585, 585, 585, 585, 585, 585, 585, 585, 585, 585, 585, 585, 585, 585, 585, 585, 585, 585, 585, 585, 585, 585, 585, 585, 585, 585, 585, 585, 585, 585, 585, 585, 585, 585, 585, 585, 585, 585, 585, 585, 585, 585, 585, 585, 585, 585, 585, 585, 585, 585, 585, 585, 585, 585, 585, 585, 585, 585, 585, 585, 585, 585]
  out "Y positions camera 1 \n(image \ncoordinates)":i32[](array[numeric])=[446, 446, 446, 445, 446, 445, 446, 446, 446, 446, 446, 445, 445, 446, 445, 446, 445, 446, 446, 446, 445, 445, 446, 446, 445, 445, 446, 445, 446, 445, 445, 445, 445, 445, 446, 446, 445, 445, 445, 446, 446, 445, 445, 445, 446, 446, 446, 445, 446, 446, 446, 446, 446, 445, 446, 446, 445, 446, 445, 446, 445, 445, 445, 446, 445, 446, 446, 446, 446, 446, 445, 445, 445, 445, 446, 445, 445, 445, 445, 446, 445, 446, 446, 446, 446, 446, 446, 445, 445, 446, 445, 445, 445, 445, 445, 445, 445, 445, 446, 446, 446, 445, 446, 445, 446, 445, 445, 446, 446, 446, 446, 445, 446, 445, 446, 445, 445, 445, 446, 446, 445, 445, 446, 445, 446, 445, 446, 446, 445, 446, 446, 445, 445, 445, 446, 445, 446, 445, 445, 446, 446, 445, 445, 446, 445, 446, 446, 446, 446, 445, 445, 446, 445, 445, 446, 445, 445, 445, 445, 445, 445, 446, 446, 445, 446, 445, 446, 446, 445, 446, 445, 446, 446, 445, 446, 446, 445, 446, 445, 446, 446, 446, 445, 446, 445, 446, 446, 445, 446, 445, 446, 445, 446, 445, 446, 445, 445, 445, 446, 445, 446, 446, 446, 445, 445, 446, 446, 446, 445, 446, 445, 446, 445, 446, 446, 446, 446, 446, 446, 446, 446, 445, 446, 445, 445, 445, 446, 445, 445, 446, 445, 445, 446, 446, 446, 445, 446, 445, 446, 446, 446, 445, 445, 445, 446, 446, 446, 445, 445, 445, 446, 445, 445, 446, 445, 445, 446, 446, 445, 445, 446, 446, 446, 446, 446, 446, 446, 446, 446, 446, 445, 446, 445, 445, 445, 446, 445, 446, 445, 446, 445, 445, 445, 446, 446, 446, 445, 446, 445, 445, 445, 446, 446, 446, 446, 445, 446, 446, 446, 445, 445, 445, 446, 446, 446, 446, 445, 446, 445, 446, 446, 445, 446, 446, 446, 446, 445, 446, 445, 445, 445, 446, 446, 445, 446, 446, 445, 446, 446, 446, 446, 446, 446, 445, 446, 446, 445, 446, 446, 445, 446, 445, 446, 446, 446, 446, 445, 446, 446, 446, 446, 446, 445, 446, 446, 446, 446, 446, 446, 446, 445, 445, 445, 445, 445, 445, 445, 446, 445, 446, 446, 446, 446, 445, 446, 446, 445, 445, 445, 445, 445, 446, 445, 445, 445, 445, 446, 446, 445, 445, 445, 445, 446, 445, 446, 446, 446, 446, 445, 445, 445, 445, 445, 446, 445, 445, 446, 445, 445, 446, 446, 446, 445, 446, 445, 446, 445, 446, 445, 446, 445, 446, 445, 446, 446, 445, 446, 445, 446, 445, 445, 446, 446, 445, 445, 445, 445, 445, 446, 445, 445, 446, 446, 446, 446, 445, 446, 445, 446, 446, 446, 445, 445, 446, 445, 446, 446, 446, 446, 445, 446, 445, 446, 446, 445, 446, 446, 445, 445, 446, 446, 445, 446, 446, 446, 445, 446, 446, 446, 445, 445, 445, 446, 445, 446, 446, 446, 446, 445, 445, 446, 445, 445, 446, 445, 446, 446, 446, 446, 446, 445]
  out "LIVE":bool
  in  "stop":bool
  out "Camera backlog":i32(slide)=-1 scale=0.0..50.0
  in  "IMAQdx Device Camera":T3="cam2"
  in  "Buffers Camera 1":u32=50
  out "Image":T4(plugin-control)
  # "PROGRAM INFO\n\nThis program finds the\nfirst pixel below the \nuser threshold in\nthe user specified\nROI below"
  # "Camera search ROI"
  # "Data acquisition \nsettings"
  # "issues\n\nHow do we know if frames \nare dropped?\n\nProbably will need to save data\nin sections to an open file\n\nCould have a sliding ROI based\non previous trailing edge position\n\nCould process each data chunk\nseparately to avoid frame dropping\nissues.  I.e. if you write every 1000\npoints, then in post processing only\nprocess 1000 at a time."
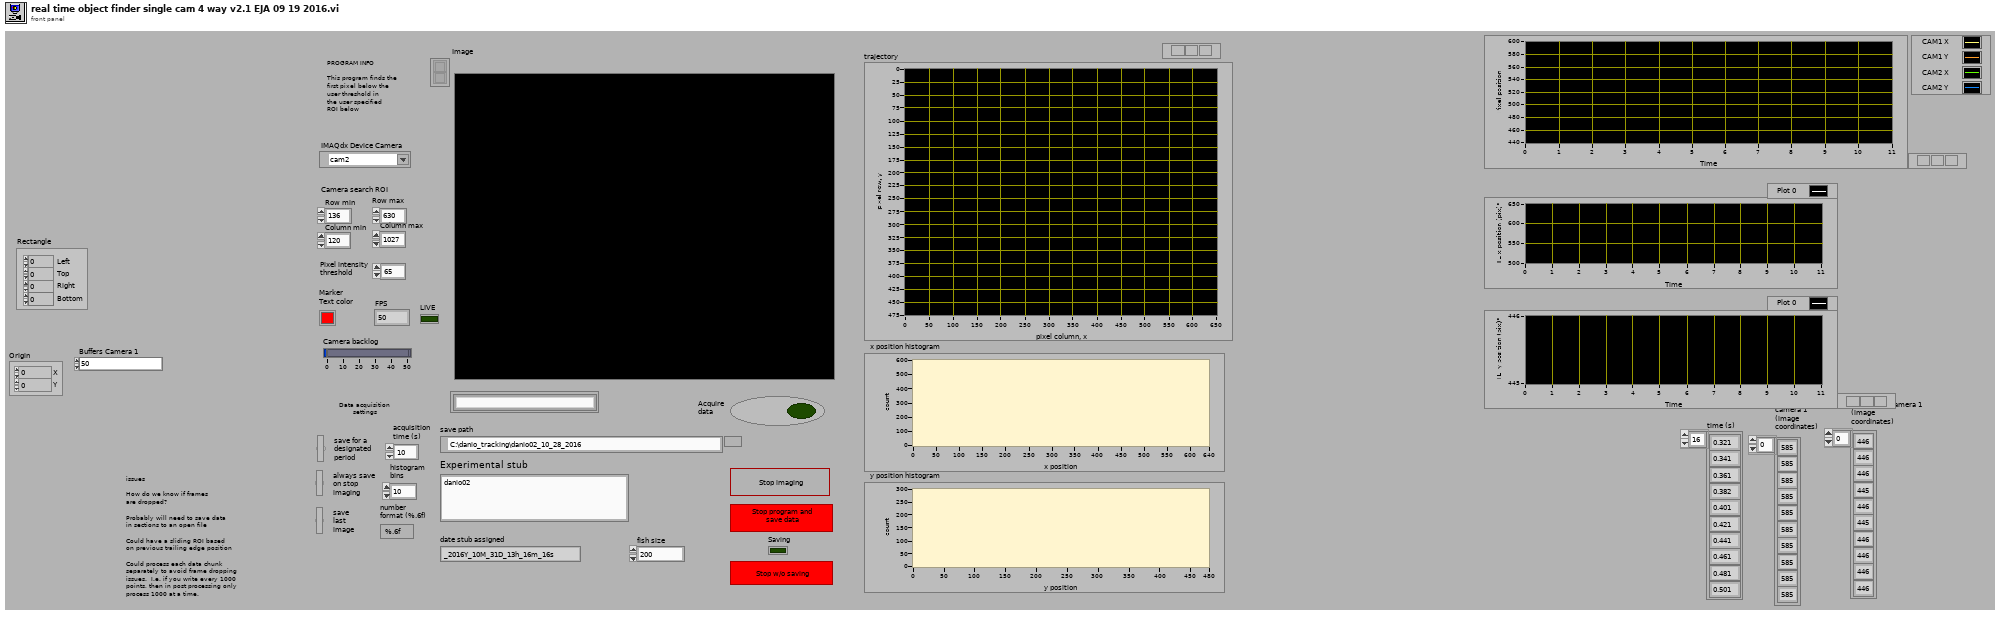
[diagram p1: front panel]
types:
  T1 = cluster{"Left":i32, "Top":i32, "Right":i32, "Bottom":i32}
  T2 = cluster{"X Values":dbl[], "Histogram: h(x)":i32[]}
  T3 = typedef "IMAQdx.ctl" = refnum<k21>
  T4 = typedef "IMAQ Image.ctl" = refnum<image>
  T5 = typedef "NI_Vision_Acquisition_Software.lvlib/IMAQdx Buffer Number Mode.ctl" = enum32{"Next", "Last", "Buffer Number"}
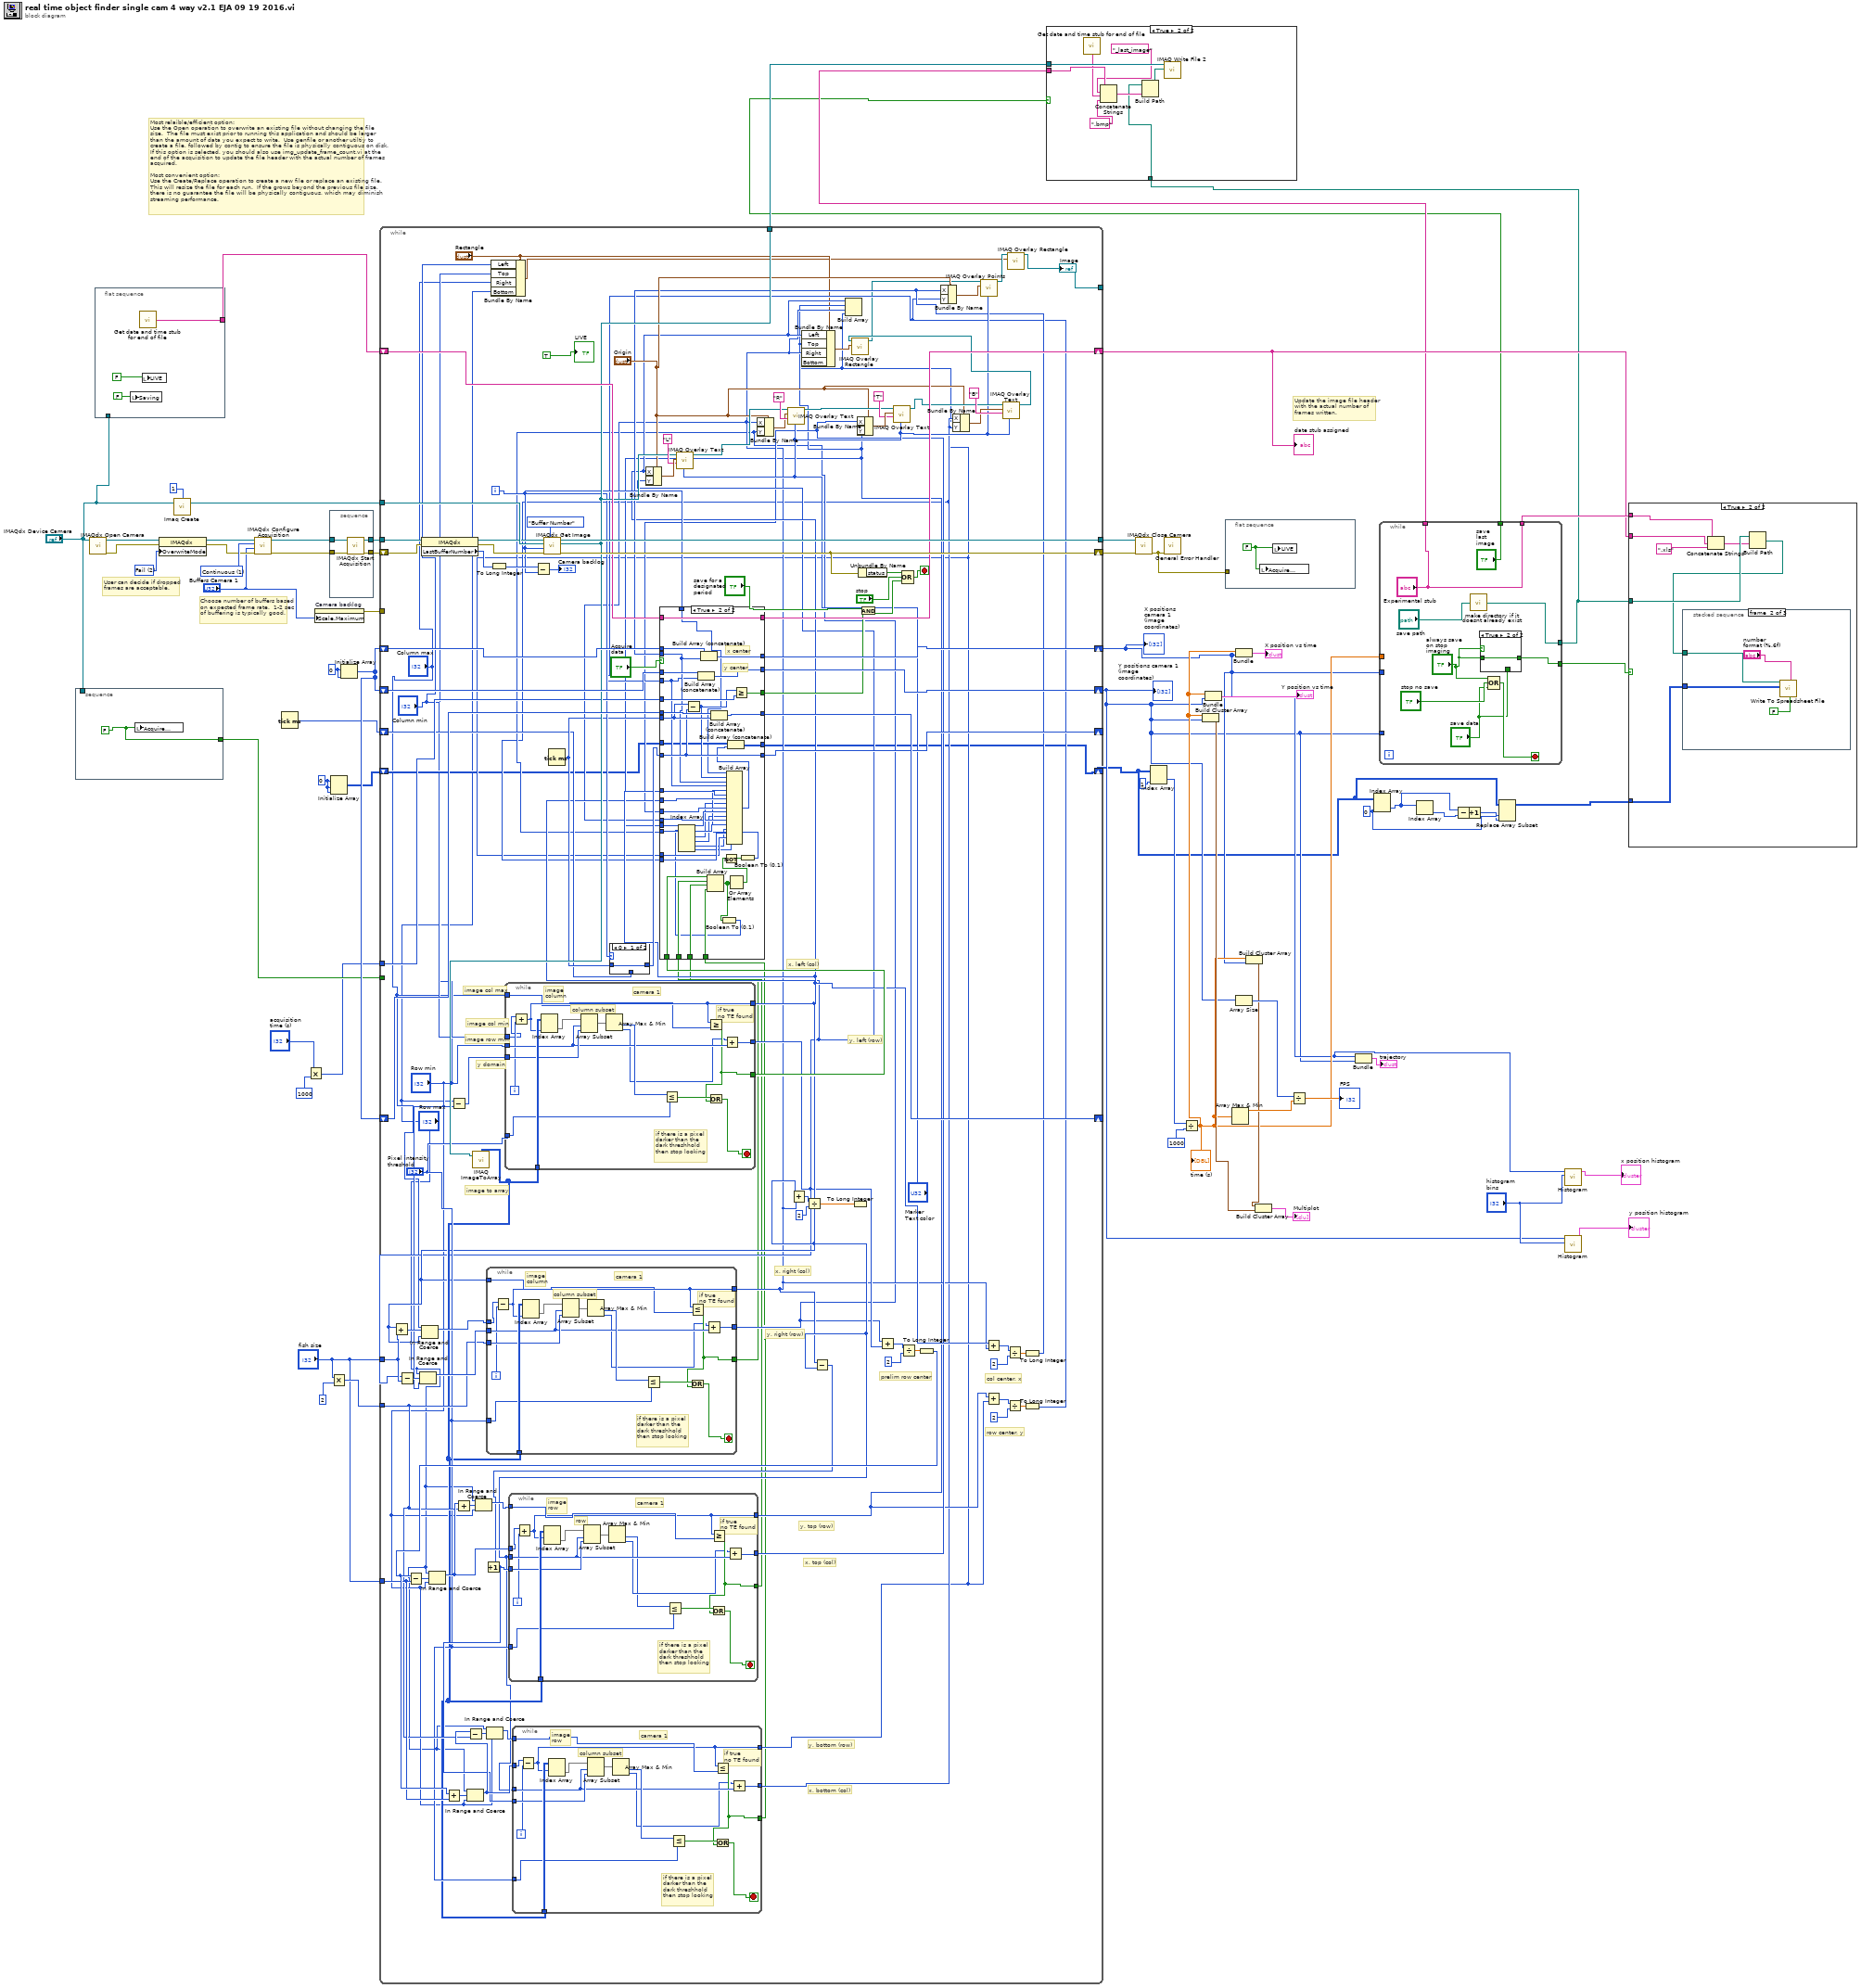
[diagram p0: block diagram]
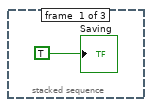
[diagram p4: hidden frame]
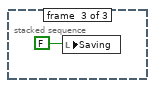
[diagram p5: hidden frame]
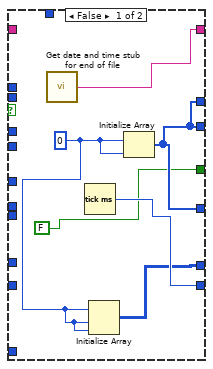
[diagram p8: hidden frame]
diagram:
  w3 = 0
  w11 = 0
  w36 = 0
  w56 = u32 2 items=["Get Oldest"=0, "Fail"=2, "Get Newest"=3] ("OverwriteMode")
  w62 = u32 1 items=["One Shot", "Continuous"] ("Continuous ?")
  # "Update the image file header with the actual number of frames written."
  # "Choose number of buffers based on expected frame rate.  1-2 sec of buffering is typically good."
  # "User can decide if dropped frames are acceptable."
  # "Most relaible/efficient option:\nUse the Open operation to overwrite an existing file without changing the file size.  The file must exist prior to running this application and should be larger than the amount of data you expect to write.  Use genfile or another utiltiy to create a file, followed by contig to ensure the file is physically contiguous on disk.  If this option is selected, you should also use img_update_frame_count.vi at the end of the acquisition to update the file header with the actual number of frames acquired. \n\nMost convenient option:\nUse the Create/Replace operation to create a new file or replace an existing file. This will resize the file for each run.  If the grows beyond the previous file size, there is no guarantee the file will be physically contiguous, which may diminish streaming performance."
  n1 = stacked-sequence {
    tunnel: "IMAQdx Device Camera" -> [_]
    tunnel: [w64] -> w26
    frame #0 {
      w64 = FALSE
      n2 = local write "Acquire\ndata"(w64) -> ()
    }
  }
  n3 = call <vilib>:"IMAQdx Open Camera.vi"("Session In"="IMAQdx Device Camera") -> ("error out"=w52:errorcluster, "Session Out"=w51:T3)  [unwired: 2 in, 7 out]
  n4 = flat-sequence {
    tunnel: "IMAQdx Device Camera" -> [_]
    tunnel: [w65] -> w35
    frame #0 {
      n5 = local write "Saving"(FALSE) -> ()
      n6 = call <userlib>:"Get date and time stub for end of file.vi"() -> ("date and time stub"=w65:string)
      n7 = local write "LIVE"(FALSE) -> ()
    }
  }
  n8 = property class="IMAQdx"(reference=w51, error in=w52, "OverwriteMode"=w56) -> (reference out=w54:T3, error out=w53:errorcluster)
  n9 = call "Imaq Create"("Border Size"=1, "Image Name"="IMAQdx Device Camera") -> ("New Image"=w63:T4)  [unwired: 2 in, 2 out]
  n10 = call <vilib>:"IMAQdx Configure Acquisition.vi"("error in"=w53, "Number of Buffers"="Buffers Camera 1", "Continuous?"=w62, "Session In"=w54) -> ("error out"=w48:errorcluster, "Session Out"=w55:T3)  [unwired: 6 out]
  n11 = Tick Count (ms)() -> (millisecond timer value=w20:u32)
  n12 = Multiply(x="acquisition \ntime (s)", y=1000) -> (x*y=w21:i32)
  n13 = property on="Camera backlog" class="Slide (strict)"("Scale.Maximum"="Buffers Camera 1") -> (error out=w50:errorcluster)  [unwired: 2 in, 1 out]
  n14 = stacked-sequence {
    tunnel: [w71] -> w61
    tunnel: [w70] -> w60
    tunnel: w55 -> [w69]
    tunnel: w48 -> [w68]
    frame #0 {
      n15 = call <vilib>:"IMAQdx Start Acquisition.vi"("error in"=w68, "Session In"=w69) -> ("error out"=w71:errorcluster, "Session Out"=w70:T3)  [unwired: 8 out]
    }
  }
  n16 = Initialize Array(w11, w11, w11) -> (w10:i32[][])
  n17 = Multiply(x="fish size", y=2) -> (x*y=w13:i32)
  n18 = Initialize Array(w36, w36) -> (w33:i32[])
  n19 = while {
    tunnel: [w174] -> w58
    tunnel: w60 -> [w177]
    tunnel: w63 -> [w175]
    tunnel: [w73] -> _
    shift-right: [w173] -> w57
    shift-left: w61 -> [w176]
    tunnel: w50 -> [_]
    shift-right: [w160] -> w19
    shift-left: w33 -> [w159]
    shift-right: [w158] -> w15
    shift-left: w33 -> [w157]
    shift-right: [w156] -> _
    shift-left: w33 -> [w155]
    shift-right: [w153] -> w34
    shift-left: w35 -> [w154]
    tunnel: [w151] -> w31
    tunnel: w26 -> [_]
    shift-right: [w150] -> _
    shift-left: w20 -> [w142]
    tunnel: w21 -> [w149]
    tunnel: "fish size" -> [w139]
    tunnel: w13 -> [w115]
    tunnel: "fish size" -> [w118]
    shift-right: [w84] -> w5
    shift-left: w10 -> [w85]
    i -> [w145]
    stop <- w179 stop-if-true
    # "x, top (col)"
    # "y, top (row)"
    # "row center, y"
    # "col center, x"
    # "y, bottom (row)"
    # "x, bottom (col)"
    # "prelim row center"
    # "x, right (col)"
    # "y, right (row)"
    # "image col min"
    # "image col max"
    # "image row min"
    # "y, left (row)"
    # "x, left (col)"
    # "y domain"
    # "image to array"
    n20 = property class="IMAQdx"(reference=w177, error in=w176) -> (reference out=w170:T3, error out=w171:errorcluster, "LastBufferNumber"=w167:u32)
    n21 = Subtract(x="Row max", y="Row min") -> (x-y=w162:i32)
    n22 = To Long Integer(number=w167) -> (32bit integer=w166:i32)
    n23 = Bundle By Name(cluster="Rectangle", "Left"="Column min", "Top"="Row min", "Right"="Column max", "Bottom"="Row max") -> (w72:T1)
    n24 = Subtract(x=w166, y=w145) -> (x-y=→"Camera backlog":i32)
    n25 = call <vilib>:"IMAQdx Get Image.vi"("Buffer Number Mode (Next)"=IMAQdx_Buffer_Number_Mode."Buffer Number", "error in"=w171, "Buffer Number In"=w145, "Image In"=w175, "Session In"=w170) -> ("error out"=w173:errorcluster, "Image Out"=w151:T4, "Session Out"=w174:T3)  [unwired: 1 in, 3 out]
    n26 = call "IMAQ ImageToArray"("Image"=w151) -> ("Image Pixels (U8)"=w110:u8[][])  [unwired: 2 in, 5 out]
    n27 = while {
      tunnel: "Row min" -> [w284]
      tunnel: [w283] -> w93
      tunnel: [w285] -> w92
      tunnel: w162 -> [w287]
      tunnel: w110 -> [w289]
      tunnel: "Column max" -> [w275]
      tunnel: "Column min" -> [w276]
      tunnel: [w280] -> w152
      tunnel: "Pixel intensity\nthreshold" -> [w278]
      i -> [w277]
      stop <- w281 stop-if-true
      # "if true\nno TE found"
      # "camera 1"
      # "if there is a pixel\ndarker than the\ndark threshhold\nthen stop looking"
      # "column subset"
      # "image\ncolumn"
      n28 = Add(x=w276, y=w277) -> (x+y=w283:i32)
      n29 = Index Array(array=w289, index (col)=w283) -> (element=w288:u8[])  [unwired: 1 in]
      n30 = Array Subset(array=w288, index=w284, length=w287) -> (w286:u8[])
      n31 = Array Max & Min(array=w286) -> (min value=w290:u8, min index (indices)=w279:i32)  [unwired: 2 out]
      n32 = Less Or Equal?(x=w290, y=w278) -> (x <= y?=w282:bool)
      n33 = Greater Or Equal?(x=w283, y=w275) -> (x >= y?=w280:bool)
      n34 = Or(x=w282, y=w280) -> (x .or. y?=w281:bool)
      n35 = Add(x=w279, y=w284) -> (x+y=w285:i32)
    }
    n36 = Add(x=w93, y=w139) -> (x+y=w141:i32)
    n37 = Subtract(x=w92, y=w139) -> (x-y=w138:i32)
    n38 = In Range and Coerce(upper limit="Row max", x=w138, lower limit="Row min") -> (coerced(x)=w137:i32)  [unwired: 1 out]
    n39 = In Range and Coerce(upper limit="Column max", x=w141, lower limit=w93) -> (coerced(x)=w140:i32)  [unwired: 1 out]
    n40 = while {
      tunnel: w137 -> [w221]
      tunnel: [w220] -> w90
      tunnel: [w222] -> w88
      tunnel: w115 -> [w224]
      tunnel: w110 -> [w226]
      tunnel: w93 -> [w212]
      tunnel: w140 -> [w213]
      tunnel: [w217] -> w82
      tunnel: "Pixel intensity\nthreshold" -> [w215]
      i -> [w214]
      stop <- w218 stop-if-true
      # "if true\nno TE found"
      # "camera 1"
      # "if there is a pixel\ndarker than the\ndark threshhold\nthen stop looking"
      # "column subset"
      # "image\ncolumn"
      n41 = Subtract(x=w213, y=w214) -> (x-y=w220:i32)
      n42 = Index Array(array=w226, index (col)=w220) -> (element=w225:u8[])  [unwired: 1 in]
      n43 = Array Subset(array=w225, index=w221, length=w224) -> (w223:u8[])
      n44 = Array Max & Min(array=w223) -> (min value=w227:u8, min index (indices)=w216:i32)  [unwired: 2 out]
      n45 = Less Or Equal?(x=w227, y=w215) -> (x <= y?=w219:bool)
      n46 = Less Or Equal?(x=w220, y=w212) -> (x <= y?=w217:bool)
      n47 = Or(x=w219, y=w217) -> (x .or. y?=w218:bool)
      n48 = Add(x=w216, y=w221) -> (x+y=w222:i32)
    }
    n49 = Tick Count (ms)() -> (millisecond timer value=w144:u32)
    n50 = case shown="0" w145 {
      tunnel: w144 -> [w228 _]
      tunnel: [w228 w229] -> w143
      tunnel: w142 -> [_ w229]
      frame 0 {
      }
      frame 1, Default {
      }
    }
    n51 = Bundle By Name(cluster="Origin", "X"=w93, "Y"=w92) -> (w164:cluster{"X":i32, "Y":i32})
    n52 = call "IMAQ Overlay Text"("Text Color (black)"="Marker\nText color", "String"="L", "Origin"=w164, "Image"=w151) -> ("Image Out"=w134:T4)  [unwired: 4 in, 3 out]
    n53 = Bundle By Name(cluster="Origin", "X"=w90, "Y"=w88) -> (w135:cluster{"X":i32, "Y":i32})
    n54 = call "IMAQ Overlay Text"("Text Color (black)"="Marker\nText color", "String"="R", "Origin"=w135, "Image"=w134) -> ("Image Out"=w121:T4)  [unwired: 4 in, 3 out]
    n55 = Add(x=w93, y=w90) -> (x+y=w133:i32)
    n56 = Divide(x=w133, y=2) -> (x/y=w131:dbl)
    n57 = Subtract(x=w90, y=w93) -> (x-y=w113:i32)
    n58 = Increment(x=w113) -> (x+1=w112:i32)
    n59 = To Long Integer(number=w131) -> ()  [unwired: 1 out]
    n60 = Unbundle By Name(w173) -> ("status"=w178:bool)
    n61 = Add(x=w88, y=w92) -> (x+y=w128:i32)
    n62 = Divide(x=w128, y=2) -> (x/y=w130:dbl)
    n63 = To Long Integer(number=w130) -> (32bit integer=w119:i32)
    n64 = Subtract(x=w119, y=w118) -> (x-y=w127:i32)
    n65 = In Range and Coerce(upper limit="Row max", x=w127, lower limit="Row min") -> (coerced(x)=w126:i32)  [unwired: 1 out]
    n66 = Add(x=w119, y=w118) -> (x+y=w120:i32)
    n67 = Add(x=w126, y=w115) -> (x+y=w125:i32)
    n68 = In Range and Coerce(upper limit="Row max", x=w120, lower limit="Row min") -> (coerced(x)=w116:i32)  [unwired: 1 out]
    n69 = Subtract(x=w116, y=w115) -> (x-y=w117:i32)
    n70 = In Range and Coerce(upper limit="Row max", x=w125, lower limit="Row min") -> (coerced(x)=w124:i32)  [unwired: 1 out]
    n71 = In Range and Coerce(upper limit="Row max", x=w117, lower limit="Row min") -> (coerced(x)=w114:i32)  [unwired: 1 out]
    n72 = while {
      tunnel: w93 -> [w206]
      tunnel: [w197] -> w89
      tunnel: [w207] -> w91
      tunnel: w112 -> [w209]
      tunnel: w110 -> [w211]
      tunnel: w124 -> [w198]
      tunnel: w126 -> [w199]
      tunnel: [w203] -> w83
      tunnel: "Pixel intensity\nthreshold" -> [w201]
      i -> [w200]
      stop <- w204 stop-if-true
      # "if true\nno TE found"
      # "camera 1"
      # "if there is a pixel\ndarker than the\ndark threshhold\nthen stop looking"
      # "row"
      # "image row"
      n73 = Add(x=w199, y=w200) -> (x+y=w197:i32)
      n74 = Index Array(array=w211, index (row)=w197) -> (element=w210:u8[])  [unwired: 1 in]
      n75 = Array Subset(array=w210, index=w206, length=w209) -> (w208:u8[])
      n76 = Array Max & Min(array=w208) -> (min value=w196:u8, min index (indices)=w202:i32)  [unwired: 2 out]
      n77 = Less Or Equal?(x=w196, y=w201) -> (x <= y?=w205:bool)
      n78 = Greater Or Equal?(x=w197, y=w198) -> (x >= y?=w203:bool)
      n79 = Or(x=w205, y=w203) -> (x .or. y?=w204:bool)
      n80 = Add(x=w202, y=w206) -> (x+y=w207:i32)
    }
    n81 = while {
      tunnel: w93 -> [w189]
      tunnel: [w180] -> w86
      tunnel: [w190] -> w87
      tunnel: w112 -> [w192]
      tunnel: w110 -> [w194]
      tunnel: w114 -> [w181]
      tunnel: w116 -> [w182]
      tunnel: [w186] -> w81
      tunnel: "Pixel intensity\nthreshold" -> [w184]
      i -> [w183]
      stop <- w187 stop-if-true
      # "if true\nno TE found"
      # "camera 1"
      # "if there is a pixel\ndarker than the\ndark threshhold\nthen stop looking"
      # "column subset"
      # "image row"
      n82 = Subtract(x=w182, y=w183) -> (x-y=w180:i32)
      n83 = Index Array(array=w194, index (row)=w180) -> (element=w193:u8[])  [unwired: 1 in]
      n84 = Array Subset(array=w193, index=w189, length=w192) -> (w191:u8[])
      n85 = Array Max & Min(array=w191) -> (min value=w195:u8, min index (indices)=w185:i32)  [unwired: 2 out]
      n86 = Less Or Equal?(x=w195, y=w184) -> (x <= y?=w188:bool)
      n87 = Less Or Equal?(x=w180, y=w181) -> (x <= y?=w186:bool)
      n88 = Or(x=w188, y=w186) -> (x .or. y?=w187:bool)
      n89 = Add(x=w185, y=w189) -> (x+y=w190:i32)
    }
    n90 = Bundle By Name(cluster="Rectangle", "Left"=w93, "Top"=w89, "Right"=w90, "Bottom"=w86) -> (w106:T1)
    n91 = Build Array(w93, w89, w90, w86) -> ()  [unwired: 1 out]
    n92 = Bundle By Name(cluster="Origin", "X"=w91, "Y"=w89) -> (w123:cluster{"X":i32, "Y":i32})
    n93 = call "IMAQ Overlay Text"("Text Color (black)"="Marker\nText color", "String"="T", "Origin"=w123, "Image"=w121) -> ("Image Out"=w107:T4)  [unwired: 4 in, 3 out]
    n94 = Bundle By Name(cluster="Origin", "X"=w87, "Y"=w86) -> (w108:cluster{"X":i32, "Y":i32})
    n95 = Add(x=w93, y=w90) -> (x+y=w105:i32)
    n96 = Add(x=w89, y=w86) -> (x+y=w100:i32)
    n97 = call "IMAQ Overlay Text"("Text Color (black)"="Marker\nText color", "String"="B", "Origin"=w108, "Image"=w107) -> ("Image Out"=w99:T4)  [unwired: 4 in, 3 out]
    n98 = call "IMAQ Overlay Rectangle"("Rectangle"=w106, "Image"=w99) -> ("Image Out"=w75:T4)  [unwired: 8 in, 1 out]
    n99 = Divide(x=w105, y=2) -> (x/y=w103:dbl)
    n100 = Divide(x=w100, y=2) -> (x/y=w102:dbl)
    n101 = To Long Integer(number=w103) -> (32bit integer=w95:i32)
    n102 = To Long Integer(number=w102) -> (32bit integer=w94:i32)
    n103 = case shown="True" "Acquire\ndata" {
      tunnel: w145 -> [_ w236]
      tunnel: w95 -> [_ w262]
      tunnel: [w234 w274] -> w160
      tunnel: w159 -> [_ w273]
      tunnel: w94 -> [_ w261]
      tunnel: [w234 w272] -> w158
      tunnel: w157 -> [_ w271]
      tunnel: w144 -> [_ w267]
      tunnel: [w234 w270] -> w156
      tunnel: w155 -> [_ w269]
      tunnel: [w235 w268] -> w153
      tunnel: w154 -> [_ w268]
      tunnel: w152 -> [_ w249]
      tunnel: w143 -> [_ w266]
      tunnel: [w233 w266] -> w150
      tunnel: w149 -> [_ w265]
      tunnel: [FALSE w264] -> w148
      tunnel: w93 -> [_ w260]
      tunnel: w92 -> [_ w259]
      tunnel: w91 -> [_ w258]
      tunnel: w89 -> [_ w257]
      tunnel: w90 -> [_ w256]
      tunnel: w88 -> [_ w255]
      tunnel: w87 -> [_ w254]
      tunnel: w86 -> [_ w253]
      tunnel: w85 -> [_ w252]
      tunnel: [w231 w250] -> w84
      tunnel: w83 -> [_ w248]
      tunnel: w82 -> [_ w247]
      tunnel: w81 -> [_ w246]
      frame False {
        w232 = 0
        n104 = call <userlib>:"Get date and time stub for end of file.vi"() -> ("date and time stub"=w235:string)
        n105 = Tick Count (ms)() -> (millisecond timer value=w233:u32)
        n106 = Initialize Array(w232, w232, w232) -> (w231:i32[][])
        n107 = Initialize Array(w232, w232) -> (w234:i32[])
      }
      frame True {
        # "y center"
        # "x center"
        n108 = Subtract(x=w267, y=w266) -> (x-y=w263:u32)
        n109 = Build Array (concatenate)(w271, w261) -> (w272:i32[])
        n110 = Build Array (concatenate)(w273, w262) -> (w274:i32[])
        n111 = Build Array(w249, w248, w247, w246) -> (w242:bool[])
        n112 = Build Array (concatenate)(w269, w267) -> (w270:u32[])
        n113 = Boolean To (0,1)(Boolean=w242) -> (0, 1=w241:i16[])
        n114 = Index Array(array=w241) -> (element #1=w240:i16, element #2=w239:i16, element #3=w238:i16, element #4=w237:i16)  [unwired: 4 in]
        n115 = Or Array Elements(Boolean array=w242) -> (logical OR=w244:bool)
        n116 = Not(x=w244) -> (.not. x?=w245:bool)
        n117 = Greater Or Equal?(x=w263, y=w265) -> (x >= y?=w264:bool)
        n118 = Boolean To (0,1)(Boolean=w245) -> (0, 1=w243:i16)
        n119 = Build Array(w236, w263, w262, w261, w243, w260, w259, w240, w258, w257, w239, w256, w255, w238, w254, w253, w237) -> (w251:u32[])
        n120 = Build Array (concatenate)(w252, w251) -> (w250:u32[][])
      }
    }
    n121 = And(x="save for a \ndesignated \nperiod", y=w148) -> (x .and. y?=w147:bool)
    n122 = Compound Arithmetic op=OR(w178, "stop", w147) -> (w179:bool)
    n123 = Bundle By Name(cluster="Origin", "X"=w95, "Y"=w94) -> (w98:cluster{"X":i32, "Y":i32})
    n124 = call "IMAQ Overlay Points"("Color"="Marker\nText color", "Point"=w98, "Image"=w75) -> ("Image Out"=w74:T4)  [unwired: 7 in, 1 out]
    n125 = call "IMAQ Overlay Rectangle"("Rectangle"=w72, "Image"=w74) -> ("Image Out"=w73:T4)  [unwired: 8 in, 1 out]
    "Image" <- w73
    "LIVE" <- TRUE
  }
  "X positions\ncamera 1\n(image \ncoordinates)" <- w19
  "Y positions camera 1 \n(image \ncoordinates)" <- w15
  "date stub assigned" <- w34
  n126 = call <vilib>:"IMAQdx Close Camera.vi"("error in"=w57, "Session In"=w58) -> ("error out"=w47:errorcluster)  [unwired: 9 out]
  n127 = Index Array(array=w5, index (col)=1) -> (element=w8:u32[])  [unwired: 1 in]
  n128 = call <vilib>:"General Error Handler.vi"("error in (no error)"=w47) -> ()  [unwired: 1 in, 14 out]
  n129 = Divide(x=w8, y=1000) -> (x/y=w25:dbl[])
  "time (s)" <- w25
  n130 = Build Cluster Array(w25, w15) -> (w38:cluster{dbl, i32}[])
  n131 = Bundle(w25, w15) -> (→"Y position vs time":cluster{dbl[], i32[]})  [unwired: 1 out]
  n132 = flat-sequence {
    tunnel: w47 -> [_]
    frame #0 {
      w291 = FALSE
      n133 = local write "Acquire\ndata"(w291) -> ()
      n134 = local write "LIVE"(w291) -> ()
    }
  }
  n135 = Array Max & Min(array=w25) -> (max value=w44:dbl)  [unwired: 3 out]
  n136 = Bundle(w25, w19) -> (→"X position vs time":cluster{dbl[], i32[]})  [unwired: 1 out]
  n137 = Array Size(array=w15) -> (size(s)=w43:i32)
  n138 = Build Cluster Array(w25, w19) -> (w39:cluster{dbl, i32}[])
  n139 = Build Cluster Array(w39, w38) -> (→"Multiplot":cluster{cluster{dbl, i32}[]}[])
  n140 = Divide(x=w43, y=w44) -> (x/y=→"FPS":dbl)
  n141 = Bundle(w19, w15) -> (→"trajectory":cluster{i32[], i32[]})  [unwired: 1 out]
  n142 = Index Array(array=w5, index (col)=w3) -> (element=w7:u32[])  [unwired: 1 in]
  n143 = while {
    tunnel: w25 -> [_]
    tunnel: w19 -> [_]
    tunnel: w15 -> [_]
    tunnel: [w292] -> w29
    tunnel: ["Experimental stub"] -> w37
    tunnel: [w295] -> w32
    tunnel: ["Experimental stub"] -> w30
    tunnel: ["save\nlast\nimage"] -> w28
    stop <- w297 stop-if-true
    n144 = call <userlib>:"make directory if it doesnt already exist.vi"("Path"="save path") -> ("created path"=w292:path)
    n145 = case shown="True" "always save\non stop\nimaging" {
      tunnel: [w301 w302] -> w295
      tunnel: "always save\non stop\nimaging" -> [_ w302]
      tunnel: "save data" -> [w301 _]
      frame False {
      }
      frame True {
      }
    }
    n146 = Compound Arithmetic op=OR("always save\non stop\nimaging", "stop no save", "save data") -> (w297:bool)
  }
  n147 = case shown="True" w28 {
    tunnel: w31 -> [_ w310]
    tunnel: w30 -> [_ w308]
    tunnel: w29 -> [_ w303]
    frame False {
    }
    frame True {
      n148 = call <userlib>:"Get date and time stub for end of file.vi"() -> ("date and time stub"=w306:string)
      n149 = Concatenate Strings(w308, "_last_image", w306, ".bmp") -> (w309:string)
      n150 = Build Path(base path=w303, name or relative path=w309) -> (appended path=w304:path)
      n151 = call-poly "IMAQ Write File 2"("File Path"=w304, "Image"=w310) -> ()  [unwired: 8 in, 2 out]
    }
  }
  n152 = Index Array(array=w7) -> (element=w6:u32)  [unwired: 1 in]
  n153 = Subtract(x=w7, y=w6) -> (x-y=w4:u32[])
  n154 = Increment(x=w4) -> (x+1=w1:u32[])
  n155 = Replace Array Subset(array=w5, new element=w1, index (col)=w3) -> (w2:u32[][])  [unwired: 1 in]
  n156 = call <vilib>:"Histogram.vi"("intervals"="histogram \nbins", "X"=w19) -> ("Histogram Graph"=→"x position histogram":T2)  [unwired: 6 in, 3 out]
  n157 = call <vilib>:"Histogram.vi"("intervals"="histogram \nbins", "X"=w15) -> ("Histogram Graph"=→"y position histogram":T2)  [unwired: 6 in, 3 out]
  n158 = case shown="True" w32 {
    tunnel: w37 -> [_ w316]
    tunnel: w29 -> [_ w315]
    tunnel: w34 -> [_ w312]
    tunnel: w2 -> [_ w311]
    frame False {
    }
    frame True {
      n159 = Concatenate Strings(w316, w312, ".xls") -> (w314:string)
      n160 = Build Path(base path=w315, name or relative path=w314) -> (appended path=w313:path)
      n161 = stacked-sequence {
        tunnel: w313 -> [_ w320 _]
        tunnel: w311 -> [_ w319 _]
        frame #0 {
          "Saving" <- TRUE
        }
        frame #1 {
          n162 = call-poly <vilib>:"Write To Spreadsheet File.vi"("transpose? (no:F)"=FALSE, "format (%d)"="number\nformat (%.6f)", "2D data"=w319, "file path (dialog if empty)"=w320) -> ()  [unwired: 4 in, 1 out]
        }
        frame #2 {
          n163 = local write "Saving"(FALSE) -> ()
        }
      }
    }
  }
